vi "JoystickShape.vi"(1 "JoystickValues":dbl[](array[numeric]), 2 "SlowSpeed":bool) -> (0 "JoystickOut":dbl[](array[numeric]))   [LabVIEW 2014]
uses:
  <vilib>/Rock Robotics/WPI/DriverStation/WPI_DriverStationRobotMode2.ctl
  Robot Global Data.vi
  Gantry/GantryGlobals.vi
  Automated Tasks/AutomationGlobals.vi
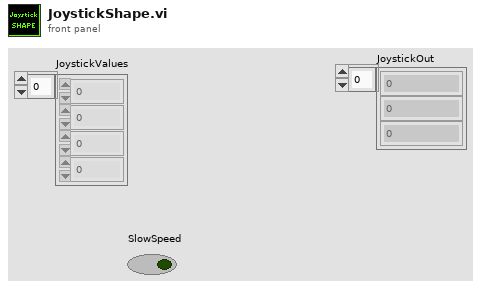
[diagram p1: front panel]
types:
  T1 = typedef "WPI_DriverStationRobotMode2.ctl" = enum16{"Autonomous Disabled", "Autonomous Enabled", "Teleop Disabled", "Teleop Enabled", "Disconnected", "Finish", "Test Disabled", "Test Enabled", "Emergency Stopped"}
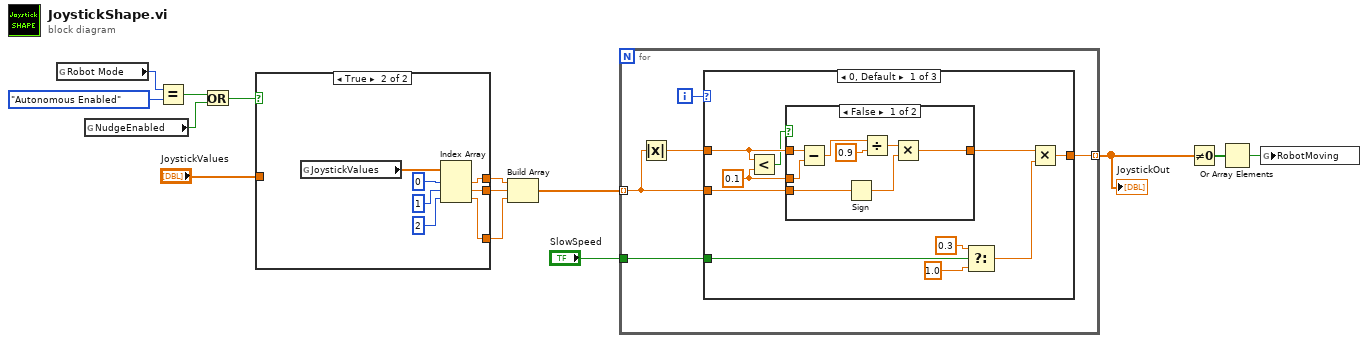
[diagram p0: block diagram]
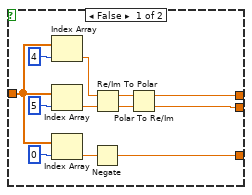
[diagram p2: hidden frame]
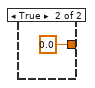
[diagram p3: hidden frame]
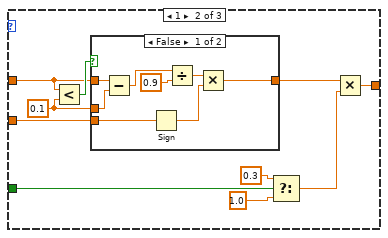
[diagram p4: hidden frame]
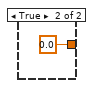
[diagram p5: hidden frame]
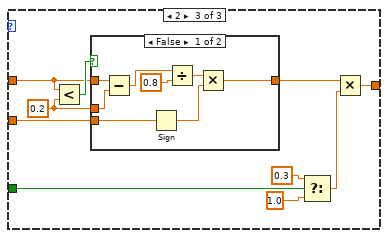
[diagram p6: hidden frame]
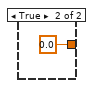
[diagram p7: hidden frame]
diagram:
  n1 = global read "Robot Global Data.vi" "Robot Mode"() -> (w10:T1)
  n2 = global read "GantryGlobals.vi" "NudgeEnabled"() -> (w7:bool)
  n3 = Equal?(x=w10, y=WPI_DriverStationRobotMode2."Autonomous Enabled") -> (x = y?=w8:bool)
  n4 = Or(x=w8, y=w7) -> (x .or. y?=w2:bool)
  n5 = case shown="True" w2 {
    tunnel: [w20 w29] -> w14
    tunnel: [w19 w28] -> w13
    tunnel: [w17 w27] -> w11
    tunnel: "JoystickValues" -> [w15 _]
    frame False {
      n6 = Index Array(array=w15, index=4) -> (element=w24:dbl)
      n7 = Index Array(array=w15, index=5) -> (element=w23:dbl)
      n8 = Index Array(array=w15, index=0) -> (element=w18:dbl)
      n9 = Negate(x=w18) -> (-x=w17:dbl)
      n10 = Re/Im To Polar(2:w23, 3:w24) -> (0:w16:dbl, 1:w22:dbl)
      n11 = Polar To Re/Im(2:w16, 3:w22) -> (0:w19:dbl, 1:w20:dbl)
    }
    frame True {
      n12 = global read "AutomationGlobals.vi" "JoystickValues"() -> (w30:dbl[])
      n13 = Index Array(array=w30, index #1=0 ("index"), index #2=1 ("index"), index #3=2 ("index")) -> (element #1=w29:dbl, element #2=w28:dbl, element #3=w27:dbl)
    }
  }
  n14 = Build Array(w14, w13, w11) -> (w12:dbl[])
  n15 = for {
    tunnel: w12 -> [w36] mode=indexing
    tunnel: [w35] -> w6 mode=indexing
    tunnel: "SlowSpeed" -> [w34]
    i -> [w38]
    n16 = Absolute Value(x=w36) -> (abs(x)=w37:dbl)
    n17 = case shown="0, Default" w38 {
      tunnel: w37 -> [w48 w66 w83]
      tunnel: [w40 w58 w78] -> w35
      tunnel: w36 -> [w46 w65 w85]
      tunnel: w34 -> [w44 w60 w77]
      frame 0, Default {
        w45 = 0.1 ("y")
        n18 = Less?(x=w48, y=w45) -> (x < y?=w47:bool)
        n19 = case shown="False" w47 {
          tunnel: w48 -> [w53 _]
          tunnel: [w55 0.0 ("y")] -> w39
          tunnel: w46 -> [w54 _]
          tunnel: w45 -> [w52 _]
          frame False {
            n20 = Subtract(x=w53, y=w52) -> (x-y=w50:dbl)
            n21 = Sign(1:w54) -> (0:w56:dbl)
            n22 = Divide(x=w50, y=0.9) -> (x/y=w49:dbl)
            n23 = Multiply(x=w49, y=w56) -> (x*y=w55:dbl)
          }
          frame True {
          }
        }
        n24 = Select(t=0.3, s=w44, f=1.0) -> (s? t:f=w43:dbl)
        n25 = Multiply(x=w39, y=w43) -> (x*y=w40:dbl)
      }
      frame 1 {
        w64 = 0.1 ("y")
        n26 = Less?(x=w66, y=w64) -> (x < y?=w67:bool)
        n27 = case shown="False" w67 {
          tunnel: w66 -> [w70 _]
          tunnel: [w68 0.0 ("y")] -> w59
          tunnel: w65 -> [w71 _]
          tunnel: w64 -> [w69 _]
          frame False {
            n28 = Subtract(x=w70, y=w69) -> (x-y=w73:dbl)
            n29 = Sign(1:w71) -> (0:w75:dbl)
            n30 = Divide(x=w73, y=0.9) -> (x/y=w72:dbl)
            n31 = Multiply(x=w72, y=w75) -> (x*y=w68:dbl)
          }
          frame True {
          }
        }
        n32 = Select(t=0.3, s=w60, f=1.0) -> (s? t:f=w63:dbl)
        n33 = Multiply(x=w59, y=w63) -> (x*y=w58:dbl)
      }
      frame 2 {
        w84 = 0.2 ("y")
        n34 = Less?(x=w83, y=w84) -> (x < y?=w86:bool)
        n35 = case shown="False" w86 {
          tunnel: [w87 0.0 ("f")] -> w79
          tunnel: w85 -> [w90 _]
          tunnel: w84 -> [w89 _]
          tunnel: w83 -> [w88 _]
          frame False {
            n36 = Subtract(x=w88, y=w89) -> (x-y=w92:dbl)
            n37 = Sign(1:w90) -> (0:w94:dbl)
            n38 = Divide(x=w92, y=0.8) -> (x/y=w91:dbl)
            n39 = Multiply(x=w91, y=w94) -> (x*y=w87:dbl)
          }
          frame True {
          }
        }
        n40 = Select(t=0.3, s=w77, f=1.0) -> (s? t:f=w82:dbl)
        n41 = Multiply(x=w79, y=w82) -> (x*y=w78:dbl)
      }
    }
  }
  "JoystickOut" <- w6
  n42 = Not Equal To 0?(x=w6) -> (x != 0?=w5:bool[])
  n43 = Or Array Elements(Boolean array=w5) -> (logical OR=w4:bool)
  n44 = global write "GantryGlobals.vi" "RobotMoving"(w4) -> ()
